vi "PiApplyPatternToAssetPreviewResponse_Parse.vi"(8 "error in (no error)":errorcluster, 11 "Message":T6) -> (0 "error out":errorcluster, 1 "Body":T1, 2 "Header":T5, 3 "PiApplyPatternToAssetPreviewResponse":T4)   [LabVIEW 2017]
uses:
  <vilib>/addons/InsightCM/MessageBus/Base/controls/Message.ctl
  <vilib>/addons/InsightCM/MessageBus/Base/controls/MessageHeader.ctl
  <vilib>/addons/InsightCM/MessageBus/Base/controls/KeyValuePair.ctl
  <vilib>/addons/InsightCM/MessageBus/MessageLibrary/PiHistorian/controls/PiApplyPatternToAssetPreviewResponse.ctl
  <vilib>/addons/InsightCM/MessageBus/MessageLibrary/PiHistorian/controls/PiApplyPatternToAssetPreviewResponseBody.ctl
  <vilib>/addons/InsightCM/MessageBus/Base/controls/PiTag.ctl
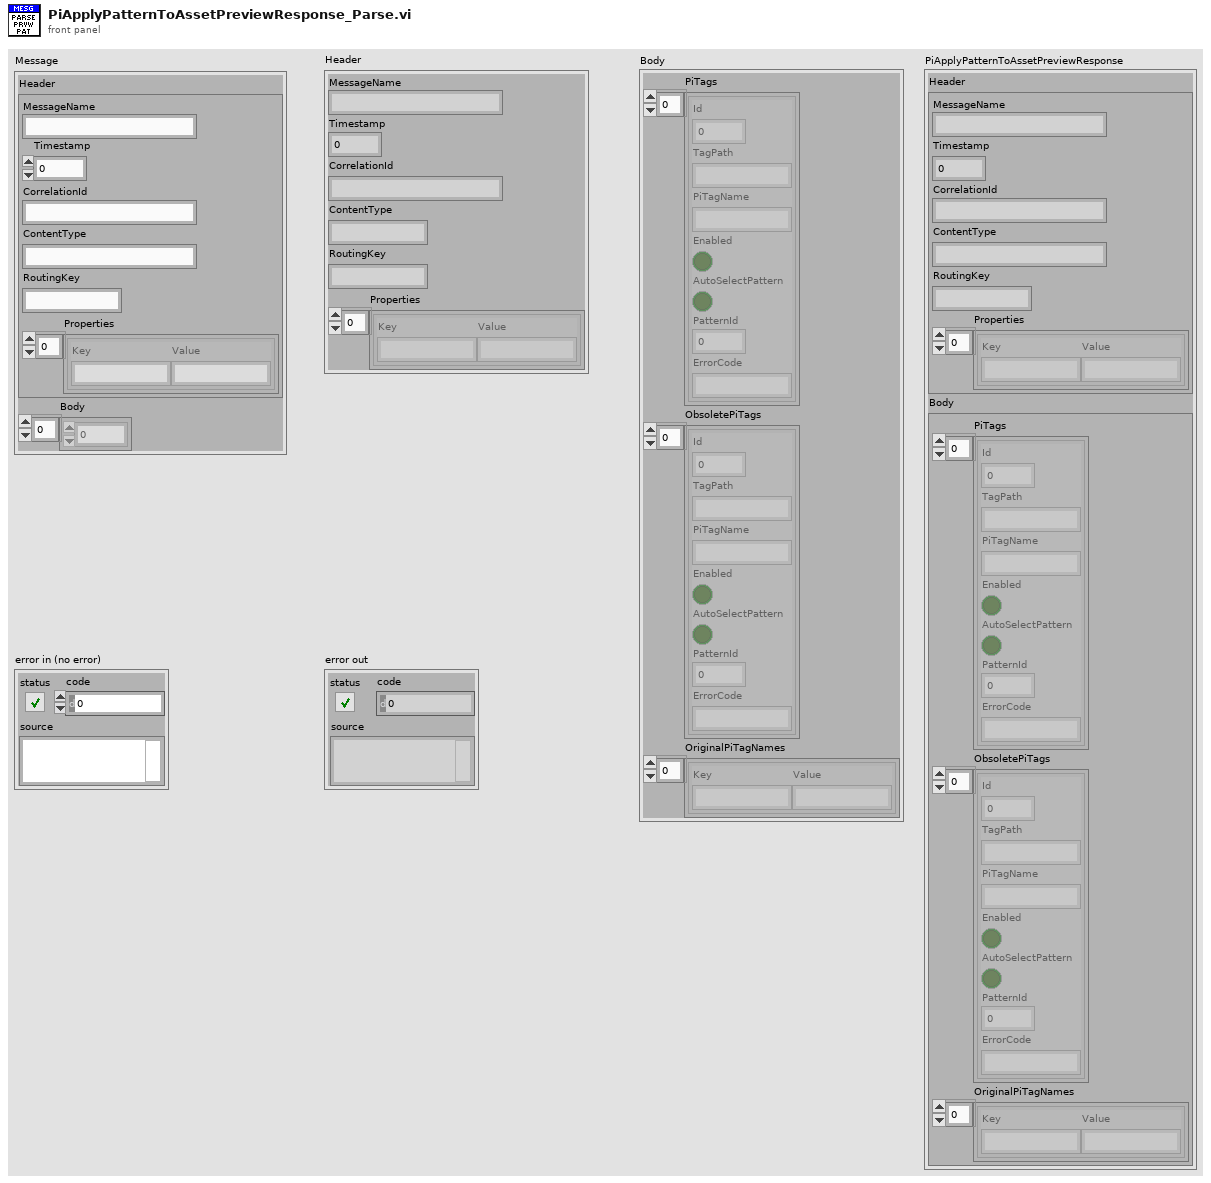
[diagram p1: front panel]
types:
  T1 = typedef "PiApplyPatternToAssetPreviewResponseBody.ctl" = cluster{"PiTags":T2[], "ObsoletePiTags":T2[], "OriginalPiTagNames":T3[]}
  T2 = typedef "PiTag.ctl" = cluster{"Id":i32, "TagPath":string, "PiTagName":string, "Enabled":bool, "AutoSelectPattern":bool, "PatternId":i32, "ErrorCode":string}
  T3 = typedef "KeyValuePair.ctl" = cluster{"Key":string, "Value":string}
  T4 = typedef "PiApplyPatternToAssetPreviewResponse.ctl" = cluster{"Header":T5, "Body":T1}
  T5 = typedef "MessageHeader.ctl" = cluster{"MessageName":string, "Timestamp":i64, "CorrelationId":string, "ContentType":string, "RoutingKey":string, "Properties":T3[]}
  T6 = typedef "Message.ctl" = cluster{"Header":T5, "Body":u8[]}
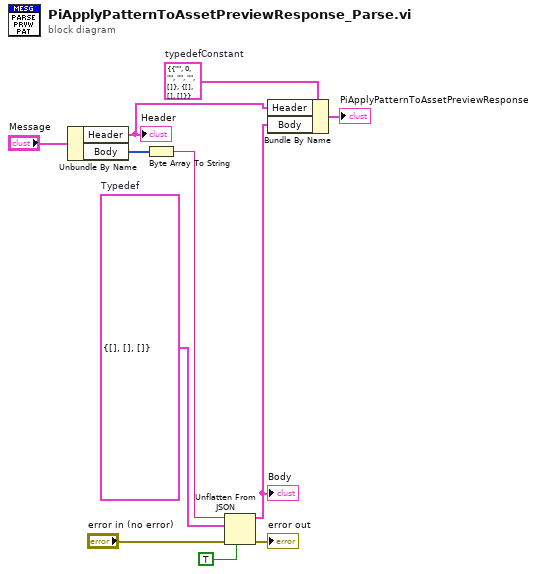
[diagram p0: block diagram]
diagram:
  w3 = T4 {"Header"={"MessageName"="", "Timestamp"=0, "CorrelationId"="", "ContentType"="", "RoutingKey"="", "Properties"=[]}, "Body"={"PiTags"=[], "ObsoletePiTags"=[], "OriginalPiTagNames"=[]}}  # typedefConstant
  w7 = T1 {"PiTags"=[], "ObsoletePiTags"=[], "OriginalPiTagNames"=[]}  # Typedef
  n1 = Unbundle By Name("Message") -> ("Header"=w9:T5, "Body"=w1:u8[])
  "Header" <- w9
  n2 = Byte Array To String(unsigned byte array=w1) -> (string=w6:string)
  n3 = Unflatten From JSON(JSON string=w6, type and defaults=w7, default null elements? (F)=TRUE, error in (no error)="error in (no error)") -> (value=w5:T1, error out=→"error out":errorcluster)  [unwired: 3 in]
  "Body" <- w5
  n4 = Bundle By Name(cluster=w3, "Header"=w9, "Body"=w5) -> (→"PiApplyPatternToAssetPreviewResponse":T4)
